vi "sweep2.vi"() -> ()   [LabVIEW 2014]
uses:
  <vilib>/measure/NI_MAPro.lvlib
  <vilib>/express/express analysis/Spectral/XNode/ExpressSpectralMeasurementsBlockNode.xnode
  <vilib>/Analysis/NI_AAL_SigProc.lvlib
  <vilib>/express/express analysis/Spectral/Block/exnSpectralBlock spectral measurements peak poly.vi
  <vilib>/express/express analysis/Spectral/Block/exnSpectralBlock spectral measurements peak DDT.vi
panel:
  out "Amplitudes":dbl[](array[numeric])
  out "Locations":dbl[](array[numeric])
  out "Waveform Graph":dynamicdata(graph)
  in  "fmin":dbl
  out "data":dynamicdata(graph)
  out "i2":dbl
  in  "tps max sec":dbl
  in  "fs":dbl
  in  "fmax":dbl
  out "resulting string":string
  in  "a":dbl
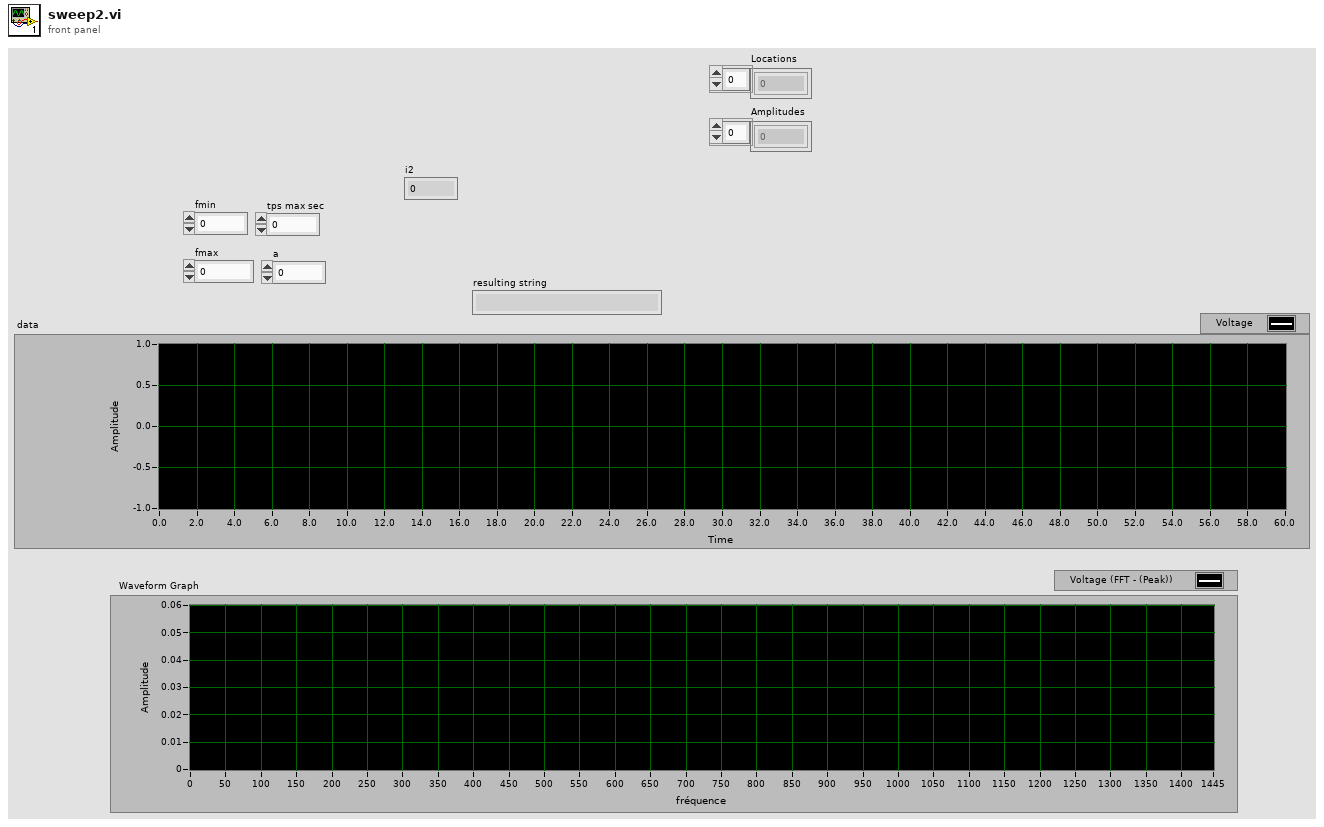
[diagram p1: front panel]
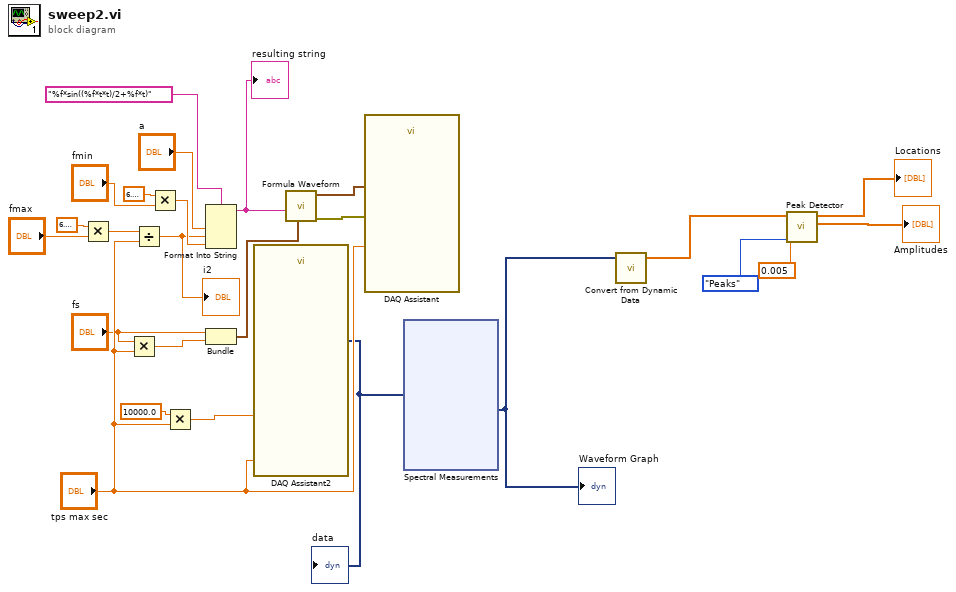
[diagram p0: block diagram]
diagram:
  n1 = Multiply(x=6.283185307179586, y="fmax") -> (x*y=w22:dbl)
  n2 = Multiply(x="fs", y="tps max sec") -> (x*y=w21:dbl)
  n3 = Divide(x=w22, y="tps max sec") -> (x/y=w12:dbl)
  "i2" <- w12
  n4 = Multiply(x=6.283185307179586, y="fmin") -> (x*y=w13:dbl)
  n5 = Multiply(x=10000.0, y="tps max sec") -> (x*y=w16:dbl)
  n6 = Format Into String(format string="%f*sin((%f*t*t)/2+%f*t)" ("signal générateur"), "a", w12, w13) -> (resulting string=w23:string)  [unwired: 2 in, 1 out]
  "resulting string" <- w23
  n7 = Bundle("fs"="fs", w21) -> (w20:cluster{"fs":dbl, dbl})  [unwired: 1 in]
  n8 = call "DAQ Assistant2"("number of samples"=w16, "timeout (s)"="tps max sec") -> ("data"=w8:dynamicdata)  [unwired: 15 in, 2 out]
  "data" <- w8
  n9 = call <vilib>:"Formula Waveform.vi"("sampling info"=w20, "formula"=w23) -> ("error out"=w18:errorcluster, "signal out"=w9:waveform(dbl))  [unwired: 8 in]
  n10 = call "DAQ Assistant"("data"=w9, "timeout (s)"="tps max sec", "error in"=w18) -> ()  [unwired: 15 in, 2 out]
  n11 = xnode "Spectral Measurements"("Signals"=w8) -> ("FFT - (Peak)"=w5:dynamicdata)  [unwired: 1 in, 2 out]
  "Waveform Graph" <- w5
  n12 = call "Convert from Dynamic Data"("Dynamic Data Type"=w5) -> ("Array"=w1:dbl[])  [unwired: 3 in]
  n13 = call <vilib>:"Peak Detector.vi"("peaks/valleys"=enum32{"Peaks", "Valleys"}."Peaks", "threshold"=0.005, "X"=w1) -> ("Amplitudes"=→"Amplitudes":dbl[], "Locations"=→"Locations":dbl[])  [unwired: 4 in, 3 out]
